vi "Replace Array Element.vi"(7 "Log?":bool, 8 "error in (no error)":errorcluster, 9 "Data":dbl, 10 "Index in":i32, 11 "Array in":dbl[][](array[numeric])) -> (0 "error out":errorcluster, 1 "Stop?":bool, 2 "Index out":i32, 3 "Array out":dbl[][](array[numeric]))   [LabVIEW 2020]
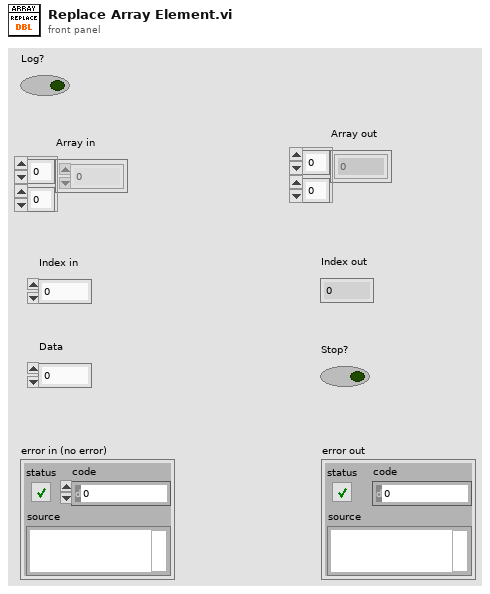
[diagram p1: front panel]
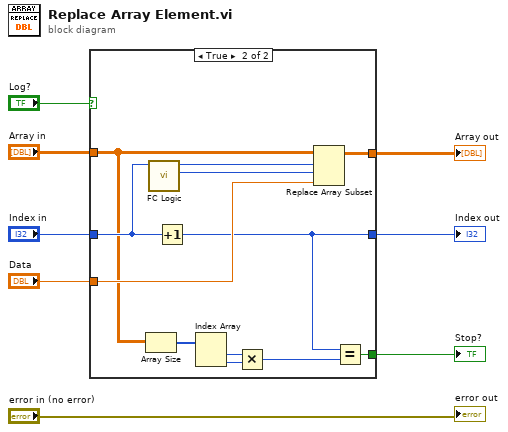
[diagram p0: block diagram]
diagram:
  n1 = case shown="True" "Log?" {
    selector: "Log?" -> [w9 _]
    tunnel: "Array in" -> [w11 w16]
    tunnel: [w11 w21] -> w4
    tunnel: "Index in" -> [w10 w20]
    tunnel: [w10 w18] -> w6
    tunnel: "Data" -> [_ w19]
    tunnel: [w9 w17] -> w8
    frame False {
    }
    frame True {
      n2 = Array Size(array=w16) -> (size(s)=w15:i32[])
      n3 = call "FC Logic.vi"("Log Iteration"=w20) -> ("Column"=w22:i32, "Row"=w23:i32)  [unwired: 9 in]
      n4 = Increment(x=w20) -> (x+1=w18:i32)
      n5 = Index Array(array=w15) -> (element #1=w13:i32, element #2=w14:i32)  [unwired: 2 in]
      n6 = Multiply(x=w13, y=w14) -> (x*y=w12:i32)
      n7 = Replace Array Subset(array=w16, new element=w19, index (row)=w23, index (col)=w22) -> (w21:dbl[][])
      n8 = Equal?(x=w18, y=w12) -> (x = y?=w17:bool)
    }
  }
  "Stop?" <- w8
  "Index out" <- w6
  "Array out" <- w4
  "error out" <- "error in (no error)"
